vi "Close Project References.vi"(0 "NI Build Specification in":refnum<class "NI Build Specification_LV.lvclass">, 11 "error in (no error)":errorcluster) -> (4 "NI Build Specification out":refnum<class "NI Build Specification_LV.lvclass">, 15 "error out":errorcluster)   [LabVIEW 2017, in "CL_G3_VIComponentBuilder.lvlib" / "NI Build Specification_LV.lvclass"]
doc: "Closes references to the project items, such as the target. Also closes all project references in sub builds.\n <MustCallParent>The parent's method is responsible for cleaning up all opened references and therefore must be called. </MustCallParent>"
uses:
  NI Build Specification_LV.lvclass
  NI Build Specification_LV.lvclass/NI Build Specification_LV.ctl
  Accessors/Read Build Spec Ref.vi
  Accessors/Read Project Reference.vi
  Accessors/Read TargetRef Containting Build Spec.vi
  Accessors/Read LabVIEW Project SubBuild Spec Order.vi
  Accessors/Write Build Spec Ref.vi
  Accessors/Write Project Reference.vi
  Accessors/Write TargetRef Containting Build Spec.vi
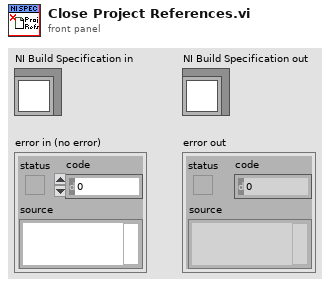
[diagram p1: front panel]
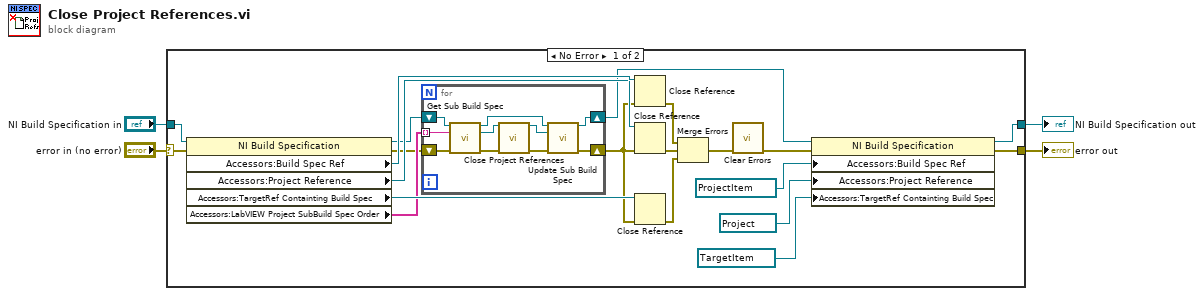
[diagram p0: block diagram]
diagram:
  n1 = case shown="No Error" "error in (no error)" {
    selector: "error in (no error)" -> [w15 w36]
    tunnel: [w7 w36] -> w3
    tunnel: [w10 w35] -> w1
    tunnel: "NI Build Specification in" -> [w16 w35]
    frame No Error {
      n2 = property class="NI Build Specification"(reference=w16, error in=w15) -> (reference out=w5:refnum<class "NI Build Specification_LV.lvclass">, error out=w8:errorcluster, "Accessors:Build Spec Ref"=w24:refnum<vi>, "Accessors:Project Reference"=w23:refnum<vi>, "Accessors:TargetRef Containting Build Spec"=w14:refnum<vi>, "Accessors:LabVIEW Project SubBuild Spec Order"=w11:string[])
      n3 = for {
        tunnel: w11 -> [w34] mode=indexing
        shift-right: [w31] -> w9
        shift-left: w8 -> [w32]
        shift-right: [w30] -> w6
        shift-left: w5 -> [w25]
        n4 = call "Get Sub Build Spec.vi"("NI Build Specification in"=w25, "Sub Build Spec Name"=w34, "error in (no error)"=w32) -> ("NI Build Specification out"=w33:refnum<class "NI Build Specification_LV.lvclass">, "Sub Build Spec"=w29:refnum<class "NI Build Specification_LV.lvclass">, "error out"=w27:errorcluster)  [unwired: 9 in, 1 out]
        n5 = call-dynamic "Close Project References.vi"("NI Build Specification in"=w29, "error in (no error)"=w27) -> ("NI Build Specification out"=w28:refnum<class "NI Build Specification_LV.lvclass">, "error out"=w26:errorcluster)  [unwired: 12 in]
        n6 = call "Update Sub Build Spec.vi"("NI Build Specification in"=w33, "Sub Build Spec"=w28, "error in (no error)"=w26) -> ("NI Build Specification out"=w30:refnum<class "NI Build Specification_LV.lvclass">, "error out"=w31:errorcluster)  [unwired: 11 in]
      }
      n7 = Close Reference(reference=w24, error in (no error)=w9) -> (error out=w20:errorcluster)
      n8 = Close Reference(reference=w23, error in (no error)=w9) -> (error out=w19:errorcluster)
      n9 = Close Reference(reference=w14, error in (no error)=w9) -> (error out=w13:errorcluster)
      n10 = Merge Errors(w20, w19, w13) -> (w18:errorcluster)
      n11 = call <vilib>:"Clear Errors.vi"("error in (no error)"=w18) -> ("error out"=w17:errorcluster)  [unwired: 5 in, 1 out]
      n12 = property class="NI Build Specification"(reference=w6, error in=w17, "Accessors:Build Spec Ref"=refnum<vi> refnum ("ref NIPKG Build Spec"), "Accessors:Project Reference"=refnum<vi> refnum ("ref project"), "Accessors:TargetRef Containting Build Spec"=refnum<vi> refnum ("TargetRef Containting Build Spec")) -> (reference out=w10:refnum<class "NI Build Specification_LV.lvclass">, error out=w7:errorcluster)
    }
    frame Error {
    }
  }
  "error out" <- w3
  "NI Build Specification out" <- w1
